vi "ArduinoTestFPorte.vi"() -> ()   [LabVIEW 2018]
uses:
  <vilib>/MakerHub/LINX/Public/Peripherals/Analog/Analog Read 1 Chan.vi
  <vilib>/MakerHub/LINX/Public/Peripherals/Analog/Analog Read N Chans.vi
  <vilib>/MakerHub/LINX/Private/Local IO/LinxAnalogRead.vi
  <vilib>/MakerHub/LINX/Public/Utilities/Check Channel.vi
  <vilib>/MakerHub/LINX/Public/Utilities/Open Serial.vi
  <vilib>/MakerHub/LINX/Private/Utilties/Generate Error.vi
  <vilib>/MakerHub/LINX/LMH-LINX.lvlib
panel:
  out "Value out":dbl
  out "Numeric":i32
  out "Average":dbl
  in  "stop":bool
  out "Under 1":dbl
  out "Over 4":dbl
  out "Voltage":dbl
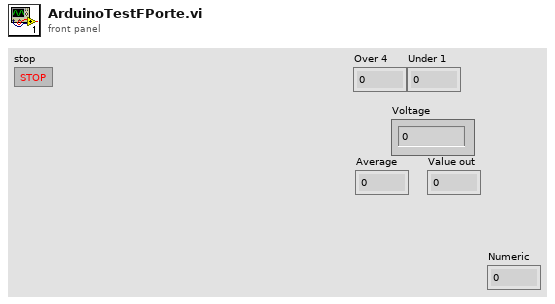
[diagram p1: front panel]
types:
  T1 = typedef "LMH-LINX.lvlib/LINX Ref.ctl" = cluster{"IO":T2, "Interface":T3, "LINX Device Config":T4}
  T2 = typedef "LMH-LINX.lvlib/Platform.ctl" = enum16{"Remote", "Local"}
  T3 = typedef "LMH-LINX.lvlib/Interface.ctl" = enum16{"Serial", "TCP"}
  T4 = typedef "LMH-LINX.lvlib/Device.lvlib/LINX Device Config.ctl" = cluster{"Interface":T3, "COM Port":refnum<visa-resource-name>, "TCP Configuration":T5, "Device Family":u8, "Device ID":u8, "Device Name":string, "TCP Ref":refnum<k5>, "Channels":T6}
  T5 = typedef "LMH-LINX.lvlib/Device.lvlib/TCP Config.ctl" = cluster{"IP Address":string, "Port":u16}
  T6 = typedef "LMH-LINX.lvlib/Channels.ctl" = cluster{"DI":u8[], "DO":u8[], "AI":u8[], "AO":u8[], "PWM":u8[], "QE":u8[], "UART":u8[], "I2C 2":u8[], "SPI":u8[], "CAN":u8[], "Servo":u8[], "AI Ref (V)":dbl, "AI Resolution (Bits)":u8, "AO Ref (V)":dbl, "AO Resolution (Bits)":u8}
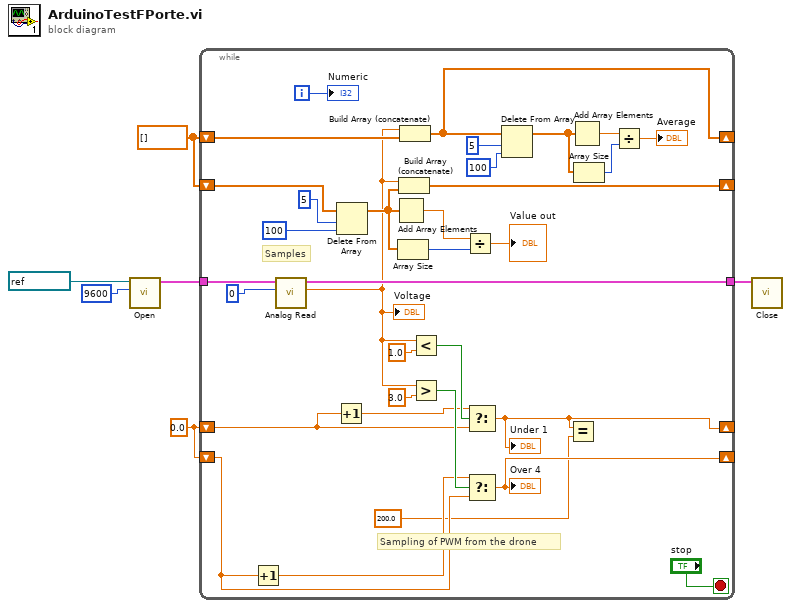
[diagram p0: block diagram]
diagram:
  w1 = dbl[] []
  w2 = 0.0
  n1 = call-poly <vilib>:"Open.vi"("Baud Rate Override"=u32 9600, "Serial Port"=refnum<visa-resource-name> "COM6") -> ("LINX Resource"=w6:T1)  [unwired: 7 in, 2 out]
  n2 = while {
    tunnel: w6 -> [w39]
    tunnel: [w38] -> w5
    shift-right: [w32] -> _
    shift-left: w2 -> [w31]
    shift-right: [w27] -> _
    shift-left: w2 -> [w29]
    shift-right: [w23] -> _
    shift-left: w1 -> [w24]
    shift-right: [w8] -> _
    shift-left: w1 -> [w9]
    i -> [w17]
    stop <- "stop" stop-if-true
    # "Sampling of PWM from the drone"
    # "Samples"
    n3 = Increment(x=w31) -> (x+1=w30:dbl)
    n4 = call-poly <vilib>:"Analog Read.vi"("Analog Channel"=u8 0, "LINX Resource"=w39) -> ("Voltage"=w7:dbl, "LINX Resource"=w38:T1)  [unwired: 6 in, 2 out]
    "Voltage" <- w7
    n5 = Increment(x=w29) -> (x+1=w28:dbl)
    n6 = Delete From Array(array=w9, length=5 ("index"), index=100 ("length")) -> (array with subset deleted=w13:dbl[])  [unwired: 1 out]
    n7 = Add Array Elements(numeric array=w13) -> (sum=w12:dbl)
    n8 = Array Size(array=w13) -> (size(s)=w14:i32)
    n9 = Build Array (concatenate)(w7, w13) -> (w8:dbl[])
    n10 = Build Array (concatenate)(w7, w24) -> (w23:dbl[])
    n11 = Less?(x=w7, y=1.0) -> (x < y?=w34:bool)
    n12 = Greater?(x=w7, y=3.0) -> (0:w33:bool)
    n13 = Divide(x=w12, y=w14) -> (x/y=→"Value out":dbl)
    n14 = Select(t=w28, s=w34, f=w29) -> (s? t:f=w27:dbl)
    "Under 1" <- w27
    n15 = Select(t=w30, s=w33, f=w31) -> (s? t:f=w32:dbl)
    "Over 4" <- w32
    n16 = Delete From Array(array=w23, length=5, index=100) -> (array with subset deleted=w21:dbl[])  [unwired: 1 out]
    n17 = Equal?(x=w27, y=200.0) -> ()  [unwired: 1 out]
    n18 = Add Array Elements(numeric array=w21) -> (sum=w20:dbl)
    n19 = Array Size(array=w21) -> (size(s)=w19:i32)
    n20 = Divide(x=w20, y=w19) -> (x/y=→"Average":dbl)
    "Numeric" <- w17
  }
  n21 = call <vilib>:"Close.vi"("LINX Resource"=w5) -> ()  [unwired: 10 in, 1 out]
